vi "Vent Status.vi"(7 "Channel (0: Channel A)":u16(ring) items=["Channel A", "Channel B"], 8 "error in (no error)":errorcluster, 11 "BH Druck PACE Series in":refnum<class "BH Druck PACE Series.lvclass">) -> (0 "error out":errorcluster, 2 "Vent Status":i32, 3 "BH Druck PACE Series out":refnum<class "BH Druck PACE Series.lvclass">)   [LabVIEW 2022 SP3, in "BH Druck PACE Series.lvclass"]
uses:
  BH Druck PACE Series.lvclass
  BH Druck PACE Series.lvclass/BH Druck PACE Series.ctl
  <vilib>/regexp/Match Regular Expression.xnode
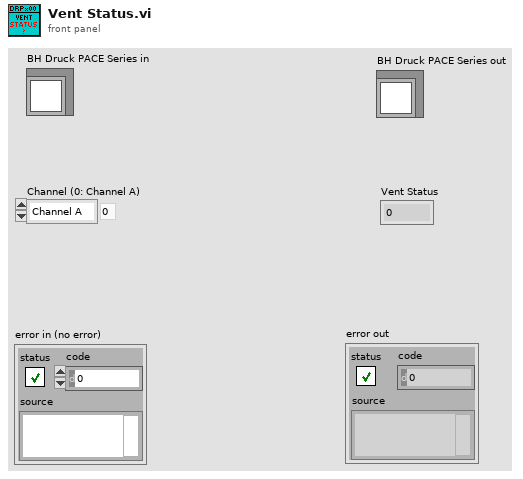
[diagram p1: front panel]
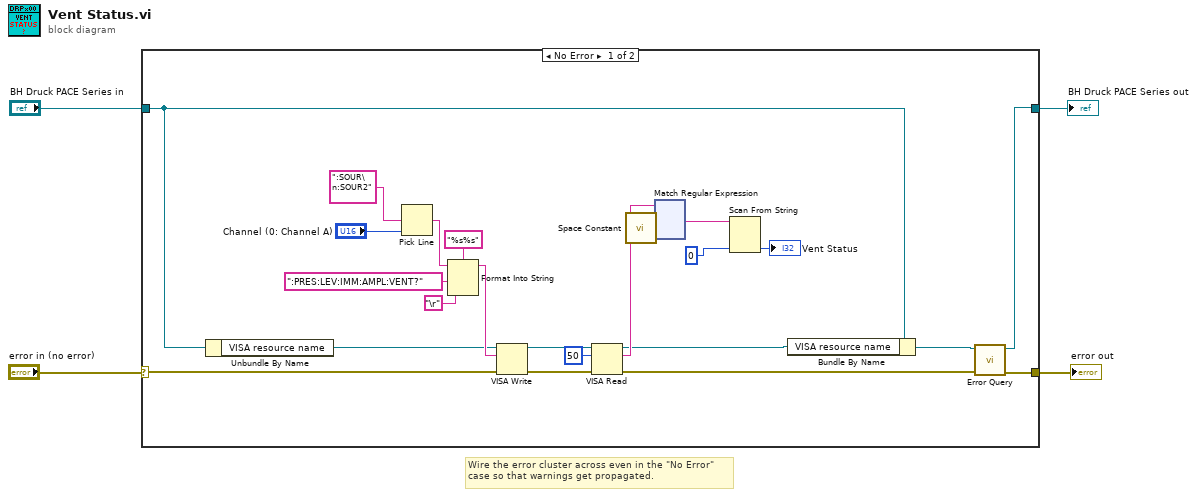
[diagram p0: block diagram]
diagram:
  # "Wire the error cluster across even in the \"No Error\"\ncase so that warnings get propagated."
  n1 = case shown="No Error" "error in (no error)" {
    selector: "error in (no error)" -> [w12 w146]
    tunnel: [w7 w146] -> w3
    tunnel: [w5 w145] -> w1
    tunnel: "BH Druck PACE Series in" -> [w10 w145]
    frame No Error {
      n2 = Unbundle By Name(w10) -> ("VISA resource name"=w9:refnum<visa-resource-name>)
      n3 = Pick Line(multi-line string=":SOUR\n:SOUR2", line index="Channel (0: Channel A)") -> (output string=w26:string)  [unwired: 1 in]
      n4 = Format Into String(format string="%s%s", initial string=w26, ":PRES:LEV:IMM:AMPL:VENT?" ("format string"), "\r") -> (resulting string=w27:string)  [unwired: 1 in, 1 out]
      n5 = VISA Write(VISA resource name=w9, write buffer=w27, error in (no error)=w12) -> (VISA resource name out=w20:refnum<visa-resource-name>, error out=w21:errorcluster)  [unwired: 1 out]
      n6 = VISA Read(VISA resource name=w20, byte count=u32 50, error in (no error)=w21) -> (VISA resource name out=w11:refnum<visa-resource-name>, read buffer=w23:string, error out=w8:errorcluster)  [unwired: 1 out]
      n7 = call <vilib>:"Space Constant.vi"() -> ("String"=w25:string)
      n8 = xnode "Match Regular Expression"("input string"=w23, "regular expression"=w25) -> ("after match"=w24:string)  [unwired: 4 in, 4 out]
      n9 = Scan From String(input string=w24, default 1=0 ("default value 1")) -> (output 1=→"Vent Status":i32)  [unwired: 3 in, 3 out]
      n10 = Bundle By Name(cluster=w10, "VISA resource name"=w11) -> (w6:refnum<class "BH Druck PACE Series.lvclass">)
      n11 = call-dynamic "Error Query.vi"("error in (no error)"=w8, "BH Druck PACE Series in"=w6) -> ("error out"=w7:errorcluster, "BH Druck PACE Series out"=w5:refnum<class "BH Druck PACE Series.lvclass">)  [unwired: 8 in]
    }
    frame Error {
    }
  }
  "error out" <- w3
  "BH Druck PACE Series out" <- w1
